vi "PQfmod.vi"(7 "error in (no error)":errorcluster, 9 "field_num":u64, 10 "res":u64) -> (0 "error out":errorcluster, 2 "modifier_type":i64, 3 "res_out":u64)   [LabVIEW 2019, in "libpqlv64.lvlib"]
doc: "Returns the type modifier of the column associated with the given column number. Column numbers start at 0.\nThe interpretation of modifier values is type-specific; they typically indicate precision or size limits. The value -1 is used to indicate \"no information available\". Most data types do not use modifiers, in which case the value is always -1."
uses:
  libpqlv64.lvlib
  libpq.dll
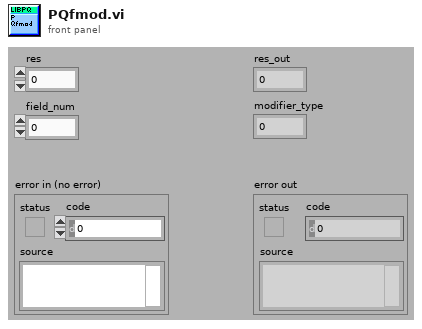
[diagram p1: front panel]
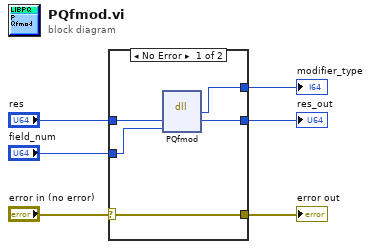
[diagram p0: block diagram]
diagram:
  n1 = case shown="No Error" "error in (no error)" {
    selector: "error in (no error)" -> [w11 w13]
    tunnel: [w11 w13] -> w5
    tunnel: [w10 _] -> w4
    tunnel: "field_num" -> [w9 _]
    tunnel: "res" -> [w8 w12]
    tunnel: [w7 w12] -> w1
    frame No Error {
      n2 = dll-call lib="libpq.*" fn="PQfmod"("res"=w8, "field_num"=w9) -> ("modifier_type"=w10:i64, "res"=w7:u64)  [unwired: 4 in, 2 out]
    }
    frame Error {
    }
  }
  "modifier_type" <- w4
  "error out" <- w5
  "res_out" <- w1
